vi "1Gear.vi"(6 "No Vision":bool, 8 "error in":errorcluster, 9 "2 Gear Side":enum16{"Left", "Right"}(ring), 10 "2 Gear":bool, 11 "Gear Side":enum16{"Center", "Left", "Right"}(ring)) -> (0 "error out":errorcluster)   [LabVIEW 2016]
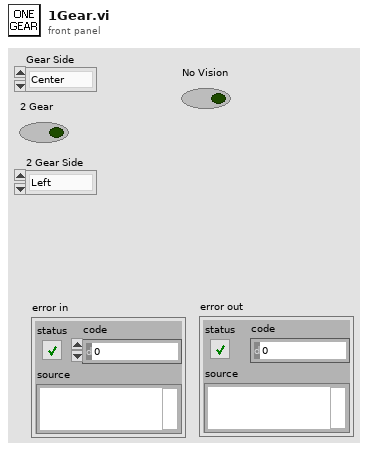
[diagram p1: front panel]
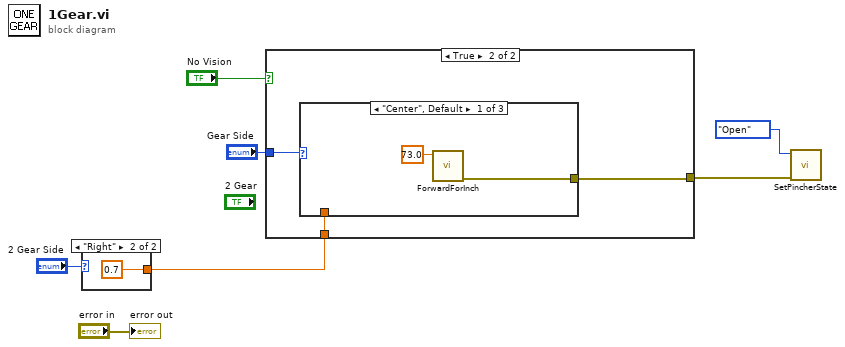
[diagram p0: block diagram]
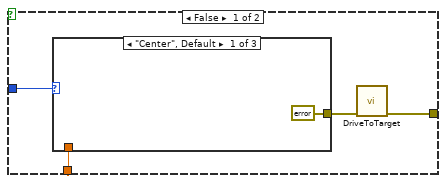
[diagram p2: hidden frame]
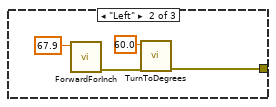
[diagram p3: hidden frame]
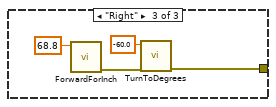
[diagram p4: hidden frame]
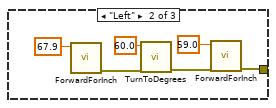
[diagram p5: hidden frame]
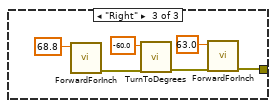
[diagram p6: hidden frame]
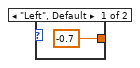
[diagram p7: hidden frame]
diagram:
  n1 = case shown="\"Right\"" "2 Gear Side" {
    tunnel: [-0.7 0.7] -> w5
    frame "Left", Default {
    }
    frame "Right" {
    }
  }
  n2 = case shown="True" "No Vision" {
    tunnel: "Gear Side" -> [w13 w25]
    tunnel: w5 -> [w12 w24]
    tunnel: [w10 w23] -> w4
    frame False {
      n3 = case shown="\"Center\", Default" w13 {
        tunnel: [errorcluster {"status"=FALSE, "code"=0, "source"=""} ("error out") w15 w19] -> w11
        tunnel: w12 -> [_ _ _]
        frame "Center", Default {
        }
        frame "Left" {
          n4 = call "ForwardForInch.vi"("Distance"=67.9) -> ("error out"=w18:errorcluster)  [unwired: 10 in]
          n5 = call "TurnToDegrees.vi"("error in"=w18, "Angle"=60.0) -> ("error out"=w15:errorcluster)  [unwired: 9 in]
        }
        frame "Right" {
          n6 = call "ForwardForInch.vi"("Distance"=68.8) -> ("error out"=w22:errorcluster)  [unwired: 10 in]
          n7 = call "TurnToDegrees.vi"("error in"=w22, "Angle"=-60.0) -> ("error out"=w19:errorcluster)  [unwired: 9 in]
        }
      }
      n8 = call "DriveToTarget.vi"("error in"=w11) -> ("error out"=w10:errorcluster)  [unwired: 10 in]
    }
    frame True {
      n9 = case shown="\"Center\", Default" w25 {
        tunnel: [w26 w29 w35] -> w23
        tunnel: w24 -> [_ _ _]
        frame "Center", Default {
          n10 = call "ForwardForInch.vi"("Distance"=73.0) -> ("error out"=w26:errorcluster)  [unwired: 10 in]
        }
        frame "Left" {
          n11 = call "ForwardForInch.vi"("Distance"=67.9) -> ("error out"=w33:errorcluster)  [unwired: 10 in]
          n12 = call "TurnToDegrees.vi"("error in"=w33, "Angle"=60.0) -> ("error out"=w30:errorcluster)  [unwired: 9 in]
          n13 = call "ForwardForInch.vi"("error in"=w30, "Distance"=59.0) -> ("error out"=w29:errorcluster)  [unwired: 9 in]
        }
        frame "Right" {
          n14 = call "ForwardForInch.vi"("Distance"=68.8) -> ("error out"=w39:errorcluster)  [unwired: 10 in]
          n15 = call "TurnToDegrees.vi"("error in"=w39, "Angle"=-60.0) -> ("error out"=w36:errorcluster)  [unwired: 9 in]
          n16 = call "ForwardForInch.vi"("error in"=w36, "Distance"=63.0) -> ("error out"=w35:errorcluster)  [unwired: 9 in]
        }
      }
    }
  }
  n17 = call "SetPincherState.vi"("error in"=w4, "PincherState"=enum16{"Open", "Close"}."Open") -> ()  [unwired: 9 in, 1 out]
  "error out" <- "error in"
